vi "String to Datafinder Comparison ENUM.vi"(11 "Modifier String":string) -> (3 "Modifier ENUM":T1)   [LabVIEW 2011]
uses:
  DataFinder Comparisons.ctl
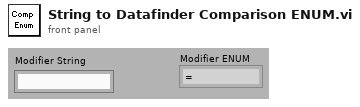
[diagram p1: front panel]
types:
  T1 = typedef "DataFinder Comparisons.ctl" = enum16{"=", "<>", "<", "<=", ">", ">="}
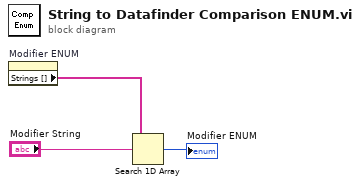
[diagram p0: block diagram]
diagram:
  n1 = property on="Modifier ENUM" class="Enum (strict)"() -> ("Strings []"=w3:string[])  [unwired: 2 in, 2 out]
  n2 = Search 1D Array(1D array=w3, element="Modifier String") -> (index of element=→"Modifier ENUM":i32)  [unwired: 1 out]
